vi "Magnification_1.vi"() -> ()   [LabVIEW 2020]
uses:
  Support/Controls/Cmd_Mouse Popup.ctl
  Support/Controls/Clst_Initialize Input.ctl
  Support/Controls/Cmd_Var Data IO.ctl
  Variables/Global_Cal Info.vi
panel:
  out "최소범위":string
  in  "눈금값":string[][](table)=[["5"], ["5"], ["5"], ["5"], ["5"], ["5"], ["5"], ["5"], ["5"], ["5"]] caption="측정 눈금값"
  out "표준자분해능":string="5" caption="표준자분해능 (mm)"
  out "단위":string
  out "최대범위":string
  in  "Spec 변경":bool
  in  "Random":bool
  out "Spec":string[][](table)
  out "제목":string
  out "에러 출력":errorcluster
  out "Condition":string[][](table) caption="2. 직선성 시험"
  in  "Measured":string[][](table) caption="측정값 (mm)"
  out "Load?":bool
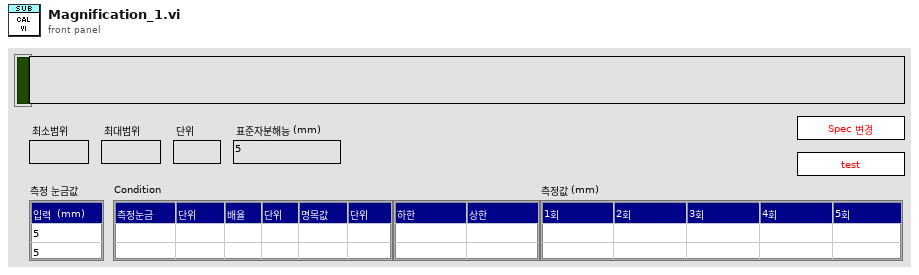
[diagram p1: front panel]
types:
  T1 = typedef "Cmd_Mouse Popup.ctl" = enum16{"활성화", "메뉴선택"}
  T2 = cluster{"Shift":bool, "Ctrl":bool, "Alt":bool, "Cmd":bool, "Opt":bool}
  T3 = typedef "Clst_Initialize Input.ctl" = cluster{"Initialize 1":cluster{"Condition":refnum<vi>[], "Spec":refnum<vi>[], "Measured":refnum<vi>[], "Resolution":refnum<vi>[], "Func_ext":string, "제목":refnum<vi>, "Measured_ADJ":refnum<vi>[]}, "Initialize 2":cluster{"문자열":refnum<vi>[], "콤보박스":refnum<vi>[], "링":refnum<vi>[], "열거형":refnum<vi>[], "테이블":refnum<vi>[], "여러열":refnum<vi>[], "디지털(DBL)":refnum<vi>[], "3D string":refnum<vi>[], "ctrl":refnum<vi>[], "boolean":refnum<vi>[]}}
  T4 = typedef "Cmd_Var Data IO.ctl" = enum16{"Condition", "Condition Default", "Condition_Temp", "Resolution", "Resolution Default", "Resolution Old", "Spec", "Spec Default", "Spec Old", "Spec Temp", "Result", "Result2", "Result3", "Result_Temp", "Result_ADJ", "Result_ADJ2", "STD1", "STD2", "STD3", "STD4", "STD5", "STD Temp", "CMC", "CMC Default"}
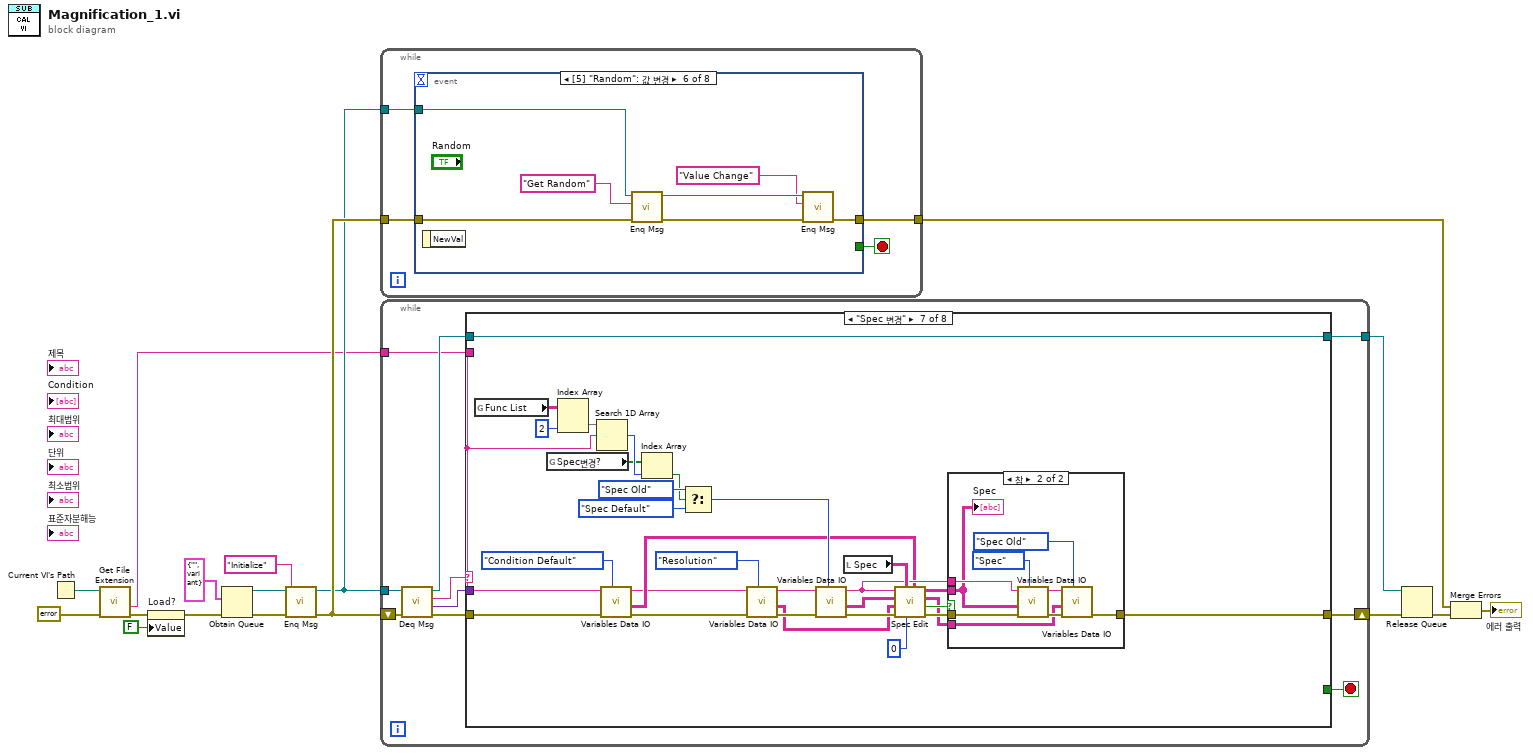
[diagram p0: block diagram]
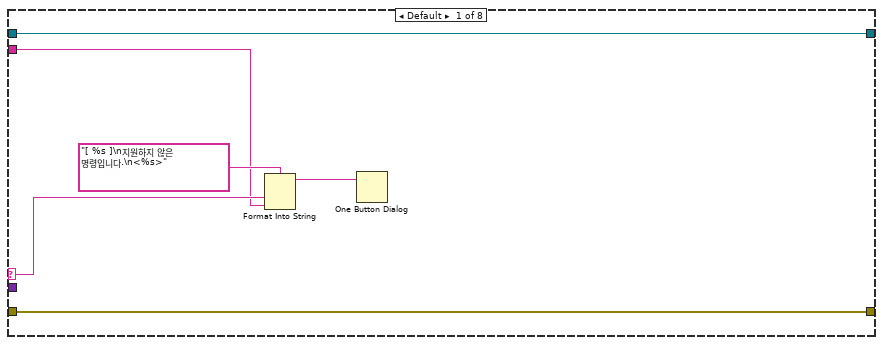
[diagram p2: hidden frame]
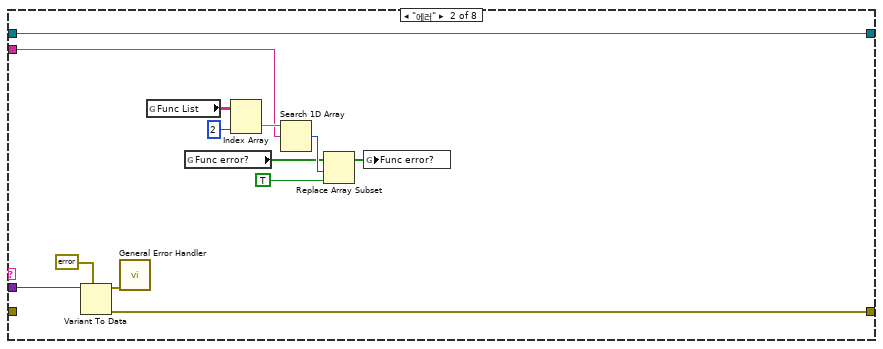
[diagram p3: hidden frame]
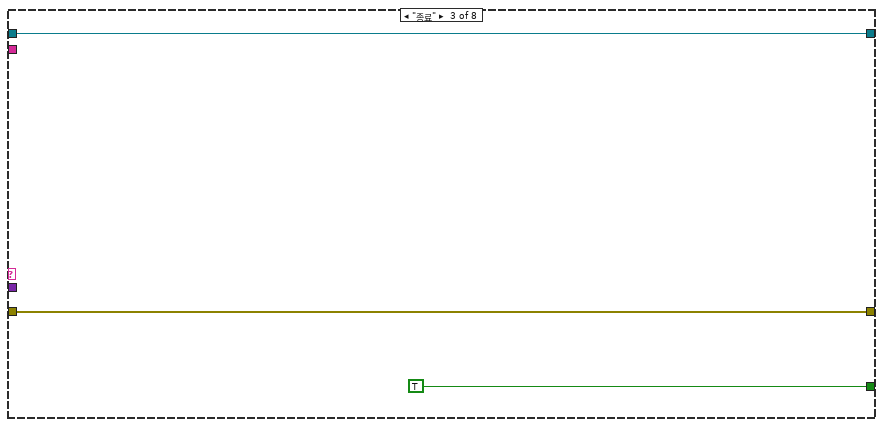
[diagram p4: hidden frame]
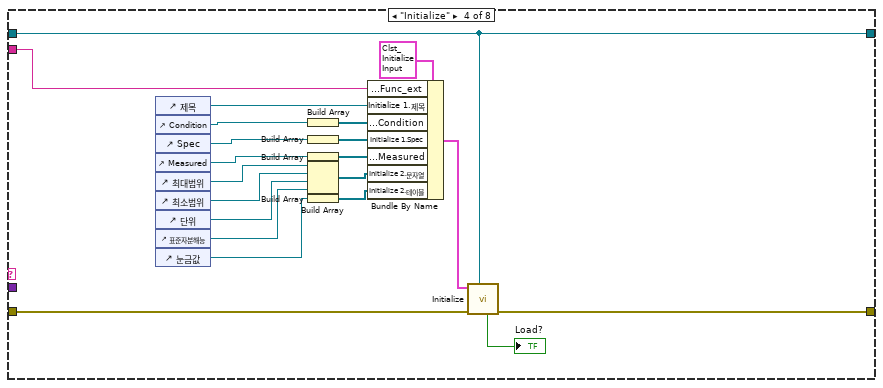
[diagram p5: hidden frame]
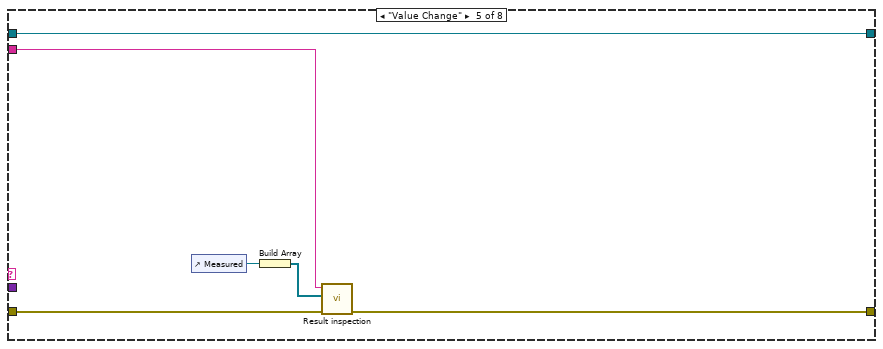
[diagram p6: hidden frame]
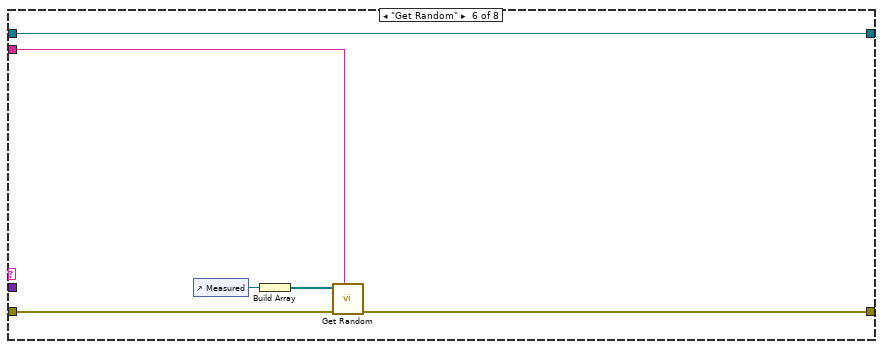
[diagram p7: hidden frame]
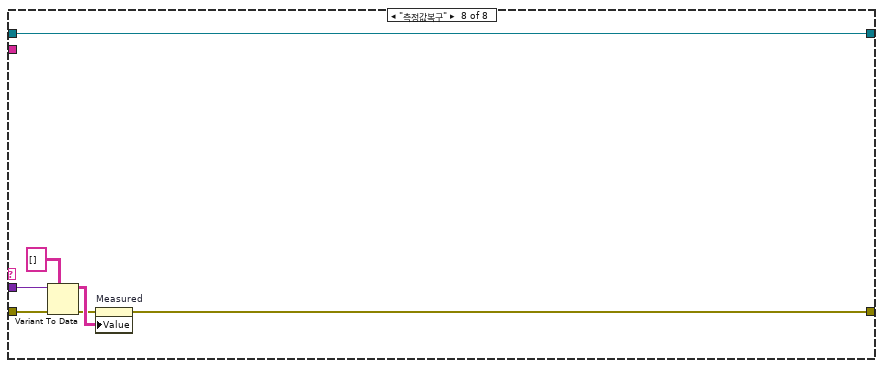
[diagram p9: hidden frame]
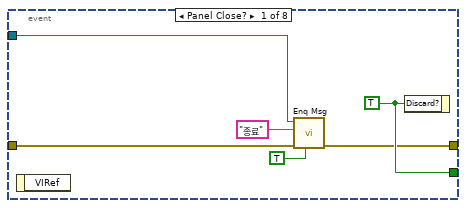
[diagram p10: hidden frame]
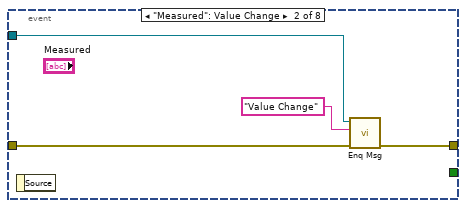
[diagram p11: hidden frame]
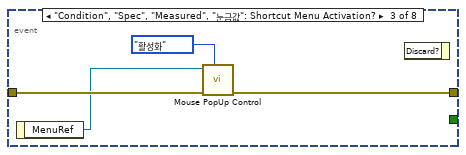
[diagram p12: hidden frame]
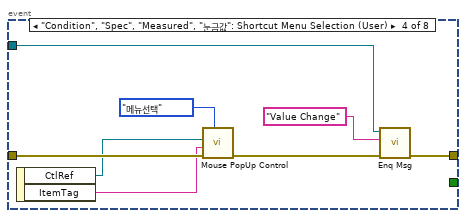
[diagram p13: hidden frame]
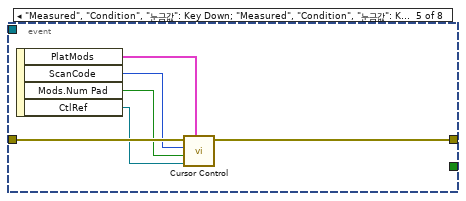
[diagram p14: hidden frame]
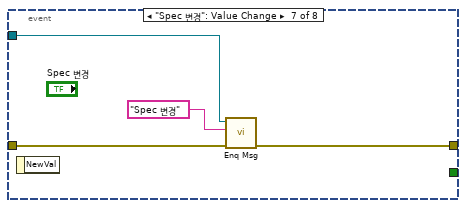
[diagram p15: hidden frame]
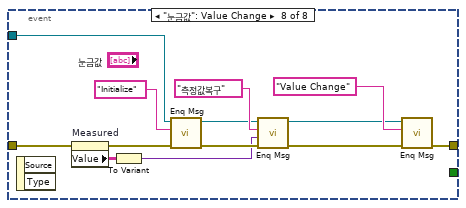
[diagram p16: hidden frame]
diagram:
  n1 = Current VI's Path() -> (path=w5:path)
  n2 = call <vilib>:"Get File Extension.vi"("error in (no error)"=errorcluster {"status"=FALSE, "code"=0, "source"=""} ("에러 상수"), "file"=w5) -> ("error out"=w3:errorcluster, "filename without extension"=w4:string)  [unwired: 5 in, 3 out]
  n3 = property on="Load?" class="Bool (엄격한)"(error in=w3, "Value"=FALSE ("Load?")) -> (error out=w2:errorcluster)  [unwired: 1 in, 1 out]
  n4 = Obtain Queue(element data type=cluster{"메세지":string, "값":variant} {"메세지"="", "값"=variant} ("Message Cluster"), error in (no error)=w2) -> (queue out=w14:refnum<queue>, error out=w16:errorcluster)  [unwired: 3 in, 1 out]
  n5 = call "Enq Msg.vi"("에러 입력(에러 없음)"=w16, "메세지"="Initialize", "큐 입력"=w14) -> ("에러 출력"=w15:errorcluster, "큐 출력"=w12:refnum<queue>)  [unwired: 7 in]
  n6 = while {
    tunnel: w15 -> [w19]
    tunnel: w12 -> [w20]
    tunnel: [w18] -> w9
    stop <- w21 stop-if-true
    n7 = event shown="[5] \"Random\": 값 변경" {
      selector: _ -> [_ _ _ _ _ _ _ _]
      dyn-events: _ -> [_ _ _ _ _ _ _ _]
      timeout: _ -> [_ _ _ _ _ _ _ _]
      tunnel: [w27 _ _ _ _ _ _ _] -> w21
      tunnel: w20 -> [w25 w31 _ w36 _ w54 w58 w72]
      tunnel: w19 -> [w26 w29 w35 w43 w49 w55 w59 w68]
      tunnel: [w23 w30 w34 w37 w48 w50 w57 w61] -> w18
      event Panel Close? {
        w27 = TRUE ("버림?")
        n8 = event-data() -> ()  [unwired: 1 in, 1 out]
        n9 = call "Enq Msg.vi"("우선순위 메시지?"=TRUE, "에러 입력(에러 없음)"=w26, "메세지"="종료", "큐 입력"=w25) -> ("에러 출력"=w23:errorcluster)  [unwired: 6 in, 1 out]
        n10 = event-data("Discard?"=w27) -> ()  [unwired: 1 in, 1 out]
      }
      event "Measured": Value Change {
        n11 = event-data() -> ()  [unwired: 1 in, 1 out]
        n12 = call "Enq Msg.vi"("에러 입력(에러 없음)"=w29, "메세지"="Value Change", "큐 입력"=w31) -> ("에러 출력"=w30:errorcluster)  [unwired: 7 in, 1 out]
      }
      event "Condition", "Spec", "Measured", "눈금값": Shortcut Menu Activation? {
        n13 = event-data() -> ("MenuRef"=w33:refnum<k9>)  [unwired: 1 in]
        n14 = call "Mouse PopUp Control.vi"("type"=Cmd_Mouse_Popup."활성화", "error in"=w35, "메뉴 참조"=w33) -> ("error out"=w34:errorcluster)  [unwired: 8 in]
        n15 = event-data() -> ()  [unwired: 2 in, 1 out]
      }
      event "Condition", "Spec", "Measured", "눈금값": Shortcut Menu Selection (User) {
        n16 = event-data() -> ("CtlRef"=w41:refnum<vi>, "ItemTag"=w40:string)  [unwired: 1 in]
        n17 = call "Mouse PopUp Control.vi"("type"=Cmd_Mouse_Popup."메뉴선택", "error in"=w43, "아이템 태그"=w40, "Tbl 참조 번호"=w41) -> ("error out"=w38:errorcluster)  [unwired: 7 in]
        n18 = call "Enq Msg.vi"("에러 입력(에러 없음)"=w38, "메세지"="Value Change", "큐 입력"=w36) -> ("에러 출력"=w37:errorcluster)  [unwired: 7 in, 1 out]
      }
      event "Measured", "Condition", "눈금값": Key Down; "Measured", "Condition", "눈금값": Key Repeat {
        n19 = event-data() -> ("PlatMods"=w44:T2, "ScanCode"=w47:i16, "Mods.Num Pad"=w46:bool, "CtlRef"=w45:refnum<vi>)  [unwired: 1 in]
        n20 = call "Cursor Control.vi"("플랫폼 조합키"=w44, "참조"=w45, "Num Pad"=w46, "ScanCode"=w47, "error in"=w49) -> ("error out"=w48:errorcluster)  [unwired: 5 in, 1 out]
      }
      event "Random": Value Change {
        n21 = event-data() -> ()  [unwired: 1 in, 1 out]
        n22 = call "Enq Msg.vi"("에러 입력(에러 없음)"=w55, "메세지"="Get Random", "큐 입력"=w54) -> ("에러 출력"=w53:errorcluster, "큐 출력"=w52:refnum<queue>)  [unwired: 7 in]
        n23 = call "Enq Msg.vi"("에러 입력(에러 없음)"=w53, "메세지"="Value Change", "큐 입력"=w52) -> ("에러 출력"=w50:errorcluster)  [unwired: 7 in, 1 out]
      }
      event "Spec 변경": Value Change {
        n24 = event-data() -> ()  [unwired: 1 in, 1 out]
        n25 = call "Enq Msg.vi"("에러 입력(에러 없음)"=w59, "메세지"="Spec 변경", "큐 입력"=w58) -> ("에러 출력"=w57:errorcluster)  [unwired: 7 in, 1 out]
      }
      event "눈금값": Value Change {
        n26 = event-data() -> ()  [unwired: 1 in, 2 out]
        n27 = property on="Measured" class="Tbl (엄격한)"(error in=w68) -> (error out=w67:errorcluster, "Value"=w66:string[][])  [unwired: 1 in, 1 out]
        n28 = To Variant(anything=w66) -> (Variant=w65:variant)
        n29 = call "Enq Msg.vi"("에러 입력(에러 없음)"=w67, "메세지"="Initialize", "큐 입력"=w72) -> ("에러 출력"=w69:errorcluster, "큐 출력"=w70:refnum<queue>)  [unwired: 7 in]
        n30 = call "Enq Msg.vi"("에러 입력(에러 없음)"=w69, "값"=w65, "메세지"="측정값복구", "큐 입력"=w70) -> ("에러 출력"=w63:errorcluster, "큐 출력"=w62:refnum<queue>)  [unwired: 6 in]
        n31 = call "Enq Msg.vi"("에러 입력(에러 없음)"=w63, "메세지"="Value Change", "큐 입력"=w62) -> ("에러 출력"=w61:errorcluster)  [unwired: 7 in, 1 out]
      }
    }
  }
  n32 = while {
    shift-right: [w83] -> w11
    shift-left: w15 -> [w82]
    tunnel: w12 -> [w80]
    tunnel: [w75] -> w10
    tunnel: w4 -> [w74]
    stop <- w76 stop-if-true
    n33 = call "Deq Msg.vi"("에러 입력(에러 없음)"=w82, "큐 입력"=w80) -> ("에러 출력"=w81:errorcluster, "값"=w77:variant, "메세지"=w79:string, "큐 출력"=w78:refnum<queue>)  [unwired: 6 in]
    n34 = case shown="\"Spec 변경\"" w79 {
      selector: w79 -> [w85 _ _ _ _ _ _ _]
      tunnel: w81 -> [w89 _ w105 w126 w129 w134 w146 w181]
      tunnel: [w89 w99 w105 w118 w131 w135 w164 w179] -> w83
      tunnel: w78 -> [w88 w98 w103 w114 w132 w138 w168 w185]
      tunnel: w77 -> [_ w100 _ _ _ _ _ w180]
      tunnel: [_ _ TRUE ("버림?") _ _ _ _ _] -> w76
      tunnel: [w88 w98 w103 w114 w132 w138 w168 w185] -> w75
      tunnel: w74 -> [w84 w90 _ w115 w130 w133 w147 _]
      frame Default {
        n35 = Format Into String(format string="[ %s ]\n지원하지 않은 명령입니다.\n<%s>" ("메시지"), w85, w84) -> (resulting string=w86:string)  [unwired: 2 in, 1 out]
        n36 = One Button Dialog(message=w86) -> ()  [unwired: 1 in, 1 out]
      }
      frame "에러" {
        n37 = Variant To Data(type=errorcluster {"status"=FALSE, "code"=0, "source"=""} ("에러 출력"), Variant=w100) -> (data=w102:errorcluster, error out=w99:errorcluster)  [unwired: 1 in]
        n38 = call <vilib>:"General Error Handler.vi"("error in (no error)"=w102) -> ()  [unwired: 10 in, 5 out]
        n39 = global read "Global_Cal Info.vi" "Func List"() -> (w92:string[][])
        n40 = global read "Global_Cal Info.vi" "Func error?"() -> (w95:bool[])
        n41 = Index Array(array=w92, index (col)=2 ("비활성화된 인덱스 (열)")) -> (element=w93:string[])  [unwired: 1 in]
        n42 = Search 1D Array(1D array=w93, element=w90) -> (index of element=w96:i32)  [unwired: 1 in]
        n43 = Replace Array Subset(array=w95, new element=TRUE ("새 원소/부분배열"), index=w96) -> (w97:bool[])
        n44 = global write "Global_Cal Info.vi" "Func error?"(w97) -> ()
      }
      frame "종료" {
      }
      frame "Initialize" {
        n45 = control-ref of="제목"() -> (w119:refnum<vi>)
        n46 = control-ref of="Condition"() -> (w123:refnum<vi>)
        n47 = control-ref of="Spec"() -> (w117:refnum<vi>)
        n48 = control-ref of="Measured"() -> (w120:refnum<vi>)
        n49 = control-ref of="최대범위"() -> (w111:refnum<vi>)
        n50 = control-ref of="최소범위"() -> (w106:refnum<vi>)
        n51 = control-ref of="단위"() -> (w113:refnum<vi>)
        n52 = control-ref of="표준자분해능"() -> (w110:refnum<vi>)
        n53 = control-ref of="눈금값"() -> (w107:refnum<vi>)
        n54 = Build Array(w123) -> (w122:refnum<vi>[])
        n55 = Build Array(w117) -> (w116:refnum<vi>[])
        n56 = Build Array(w120) -> (w121:refnum<vi>[])
        n57 = Build Array(w111, w106, w113, w110) -> (w112:refnum<vi>[])
        n58 = Build Array(w107) -> (w109:refnum<vi>[])
        n59 = Bundle By Name(cluster=T3 {"Initialize 1"={"Condition"=[], "Spec"=[], "Measured"=[], "Resolution"=[], "Func_ext"="", "제목"=refnum, "Measured_ADJ"=[]}, "Initialize 2"={"문자열"=[], "콤보박스"=[], "링"=[], "열거형"=[], "테이블"=[], "여러열"=[], "디지털(DBL)"=[], "3D string"=[], "ctrl"=[], "boolean"=[]}} ("입력 클러스터"), "Initialize 1.Func_ext"=w115, "Initialize 1.제목"=w119, "Initialize 1.Condition"=w122, "Initialize 1.Spec"=w116, "Initialize 1.Measured"=w121, "Initialize 2.문자열"=w112, "Initialize 2.테이블"=w109) -> (w124:T3)
        n60 = call "Initialize.vi"("큐 입력"=w114, "error in"=w126, "입력 클러스터"=w124) -> ("error out"=w118:errorcluster, "Load?"=→"Load?":bool)  [unwired: 5 in, 2 out]
      }
      frame "Value Change" {
        n61 = control-ref of="Measured"() -> (w128:refnum<vi>)
        n62 = Build Array(w128) -> (w127:refnum<vi>[])
        n63 = call "Result inspection.vi"("error in"=w129, "Ref. Data (Inspection)"=w127, "Func ext"=w130) -> ("error out"=w131:errorcluster)  [unwired: 5 in, 3 out]
      }
      frame "Get Random" {
        n64 = control-ref of="Measured"() -> (w137:refnum<vi>)
        n65 = Build Array(w137) -> (w136:refnum<vi>[])
        n66 = call "Get Random.vi"("Func_Ext"=w133, "에러 입력"=w134, "Meas"=w136) -> ("에러 출력"=w135:errorcluster)  [unwired: 7 in, 1 out]
      }
      frame "Spec 변경" {
        n67 = global read "Global_Cal Info.vi" "Func List"() -> (w154:string[][])
        n68 = global read "Global_Cal Info.vi" "Spec변경?"() -> (w150:bool[])
        n69 = Index Array(array=w154, index (col)=2 ("비활성화된 인덱스 (열)")) -> (element=w152:string[])  [unwired: 1 in]
        n70 = Search 1D Array(1D array=w152, element=w147) -> (index of element=w151:i32)  [unwired: 1 in]
        n71 = call "Variables Data IO.vi"("Select"=Cmd_Var_Data_IO."Condition Default", "error in"=w146, "Func_ext"=w147) -> ("error out"=w142:errorcluster, "Data Out"=w145:string[][], "Func_ext Out"=w144:string)  [unwired: 6 in]
        n72 = Index Array(array=w150, index=w151) -> (element=w155:bool)
        n73 = Select(t=Cmd_Var_Data_IO."Spec Old" ("Select"), s=w155, f=Cmd_Var_Data_IO."Spec Default" ("Select")) -> (s? t:f=w149:T4)
        n74 = call "Variables Data IO.vi"("Select"=Cmd_Var_Data_IO."Resolution", "error in"=w142, "Func_ext"=w144) -> ("error out"=w141:errorcluster, "Data Out"=w139:string[][], "Func_ext Out"=w143:string)  [unwired: 6 in]
        n75 = call "Variables Data IO.vi"("Select"=w149, "error in"=w141, "Func_ext"=w143) -> ("error out"=w163:errorcluster, "Data Out"=w158:string[][], "Func_ext Out"=w159:string)  [unwired: 6 in]
        n76 = local read "Spec"() -> (w160:string[][])
        n77 = call "Spec Edit.vi"("Condition"=w145, "열번호(기준값)"=0, "Spec Value"=w160, "에러 입력(에러 없음)"=w163, "Resolution"=w139, "Spec Default"=w158, "Func_ext"=w159) -> ("에러 출력"=w165:errorcluster, "변경?"=w166:bool, "Spec Default out"=w162:string[][], "Spec 출력"=w167:string[][])  [unwired: 1 in]
        n78 = case shown="참" w166 {
          tunnel: w167 -> [_ w175]
          tunnel: w165 -> [w169 w178]
          tunnel: [w169 w173] -> w164
          tunnel: w159 -> [_ w176]
          tunnel: w162 -> [_ w171]
          frame False {
          }
          frame True {
            n79 = call "Variables Data IO.vi"("Select"=Cmd_Var_Data_IO."Spec", "error in"=w178, "Data In"=w175, "Func_ext"=w176) -> ("error out"=w174:errorcluster, "Func_ext Out"=w172:string)  [unwired: 5 in, 1 out]
            n80 = call "Variables Data IO.vi"("Select"=Cmd_Var_Data_IO."Spec Old", "error in"=w174, "Data In"=w171, "Func_ext"=w172) -> ("error out"=w173:errorcluster)  [unwired: 5 in, 2 out]
            "Spec" <- w175
          }
        }
      }
      frame "측정값복구" {
        n81 = Variant To Data(error in=w181, type=string[][] [], Variant=w180) -> (data=w184:string[][], error out=w183:errorcluster)
        n82 = property on="Measured" class="Tbl (엄격한)"(error in=w183, "Value"=w184) -> (error out=w179:errorcluster)  [unwired: 1 in, 1 out]
      }
    }
  }
  n83 = Release Queue(queue=w10, error in (no error)=w11) -> (error out=w8:errorcluster)  [unwired: 1 in, 2 out]
  n84 = Merge Errors(w9, w8) -> (→"에러 출력":errorcluster)
